vi "Three Button Dialog CORE.vi"(4 "Allow user to close window? (TRUE)":bool=TRUE caption="Darf Anwender das Fenster schließen? (WAHR)", 5 "Justify Message (Left)":enum16{"Left", "Center", "Right"}(ring) caption="Nachricht ausrichten (Links)", 6 "Keyboard Shortcuts (Left is <Enter>)":T1={"Left Button Key Shortcut"={"Control"=FALSE, "Shift"=FALSE, "Key"="<Enter>"}, "Center Button Key Shortcut"={"Control"=FALSE, "Shift"=FALSE, "Key"=""}, "Right Button Key Shortcut"={"Control"=FALSE, "Shift"=FALSE, "Key"=""}} caption="Tastenkombimationen (Links ist <Enter>)", 7 "Window Title (\"\")":string caption="Fenstertitel (\"\")", 8 "Right Button Text (\"Cancel\")":string="Abbrechen" caption="Text der rechten Schaltfläche (\"Abbrechen\")", 9 "Center Button Text (\"No\")":string="Nein" caption="Text für mittlere Maustaste (\"No\")", 10 "Left Button Text (\"Yes\")":string="Ja" caption="Text der linken Maustaste (\"Yes\")", 11 "message":string caption="Meldung") -> (3 "Which Button?":T2(ring)=enum."Center Button" caption="Welche Schaltfläche?")   [LabVIEW 2009]
doc: "Zeigt den Text in einem Dialog mit drei Schaltflächen an. Der Enum Ausgang gibt an welche der drei Schaltflächen ausgewählt wurde oder ob der Dialog ohne Auswahl abgebrochen wurde."
panel:
  in  "OK":string="OK"
  out "C-Message":string caption="C-Nachricht"
  in  "Right Button":bool caption="Rechte Schaltfläche"
  in  "Center Button":bool caption="Mittlere Schaltfläche"
  in  "Left Button":bool caption="Linke Schaltfläche"
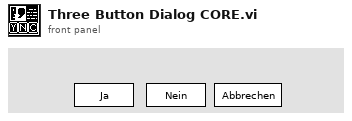
[diagram p1: front panel]
types:
  T1 = cluster{"Left Button Key Shortcut":cluster{"Control":bool, "Shift":bool, "Key":string}, "Center Button Key Shortcut":cluster{"Control":bool, "Shift":bool, "Key":string}, "Right Button Key Shortcut":cluster{"Control":bool, "Shift":bool, "Key":string}}
  T2 = enum16{"Left Button", "Center Button", "Right Button", "Window Close"}
  T3 = cluster{"left":i16, "top":i16, "right":i16, "bottom":i16}
  T4 = cluster{"Control":bool, "Shift":bool, "Key":string}
  T5 = typedef "LVRectTypeDef.ctl" = cluster{"left":i16, "top":i16, "right":i16, "bottom":i16}
  T6 = typedef "LVPointTypeDef.ctl" = cluster{"Horizontal":i16, "Vertical":i16}
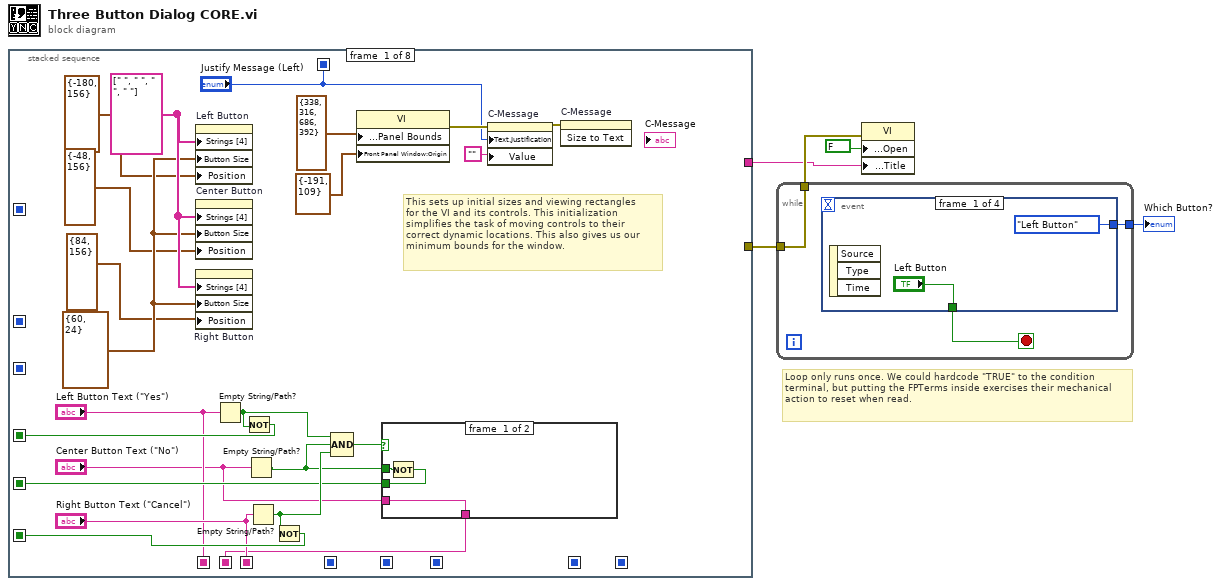
[diagram p0: block diagram]
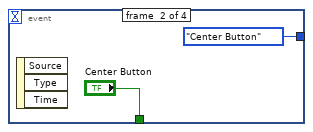
[diagram p2: hidden frame]
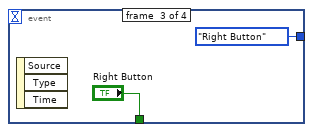
[diagram p3: hidden frame]
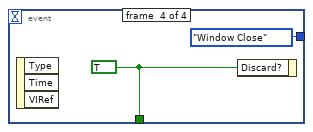
[diagram p4: hidden frame]
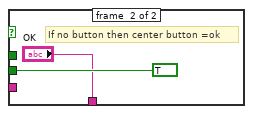
[diagram p5: hidden frame]
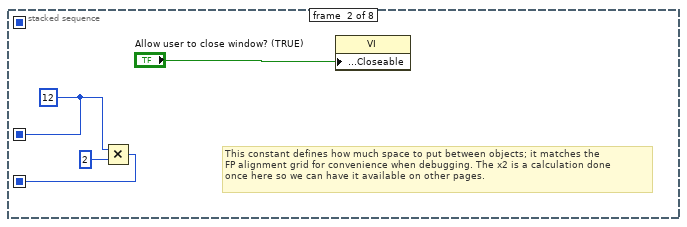
[diagram p6: hidden frame]
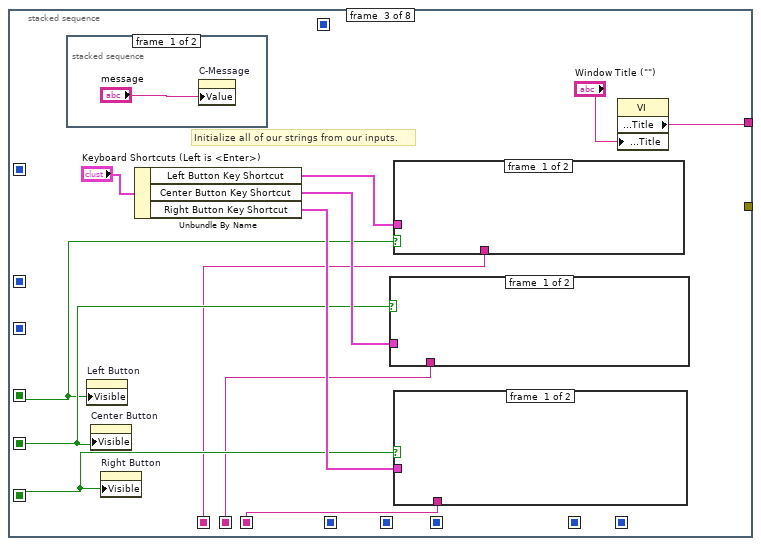
[diagram p7: hidden frame]
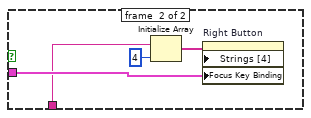
[diagram p8: hidden frame]
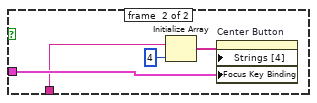
[diagram p9: hidden frame]
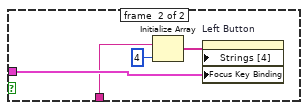
[diagram p10: hidden frame]
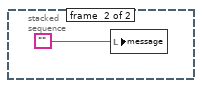
[diagram p11: hidden frame]
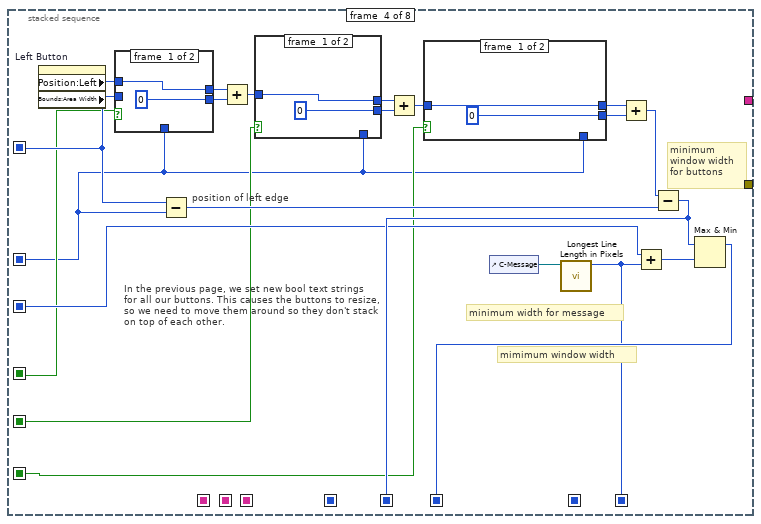
[diagram p12: hidden frame]
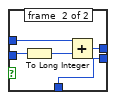
[diagram p13: hidden frame]
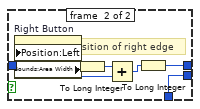
[diagram p14: hidden frame]
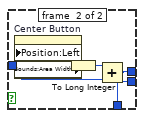
[diagram p15: hidden frame]
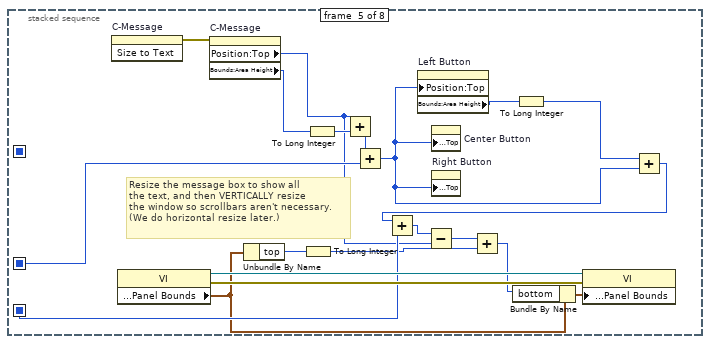
[diagram p16: hidden frame]
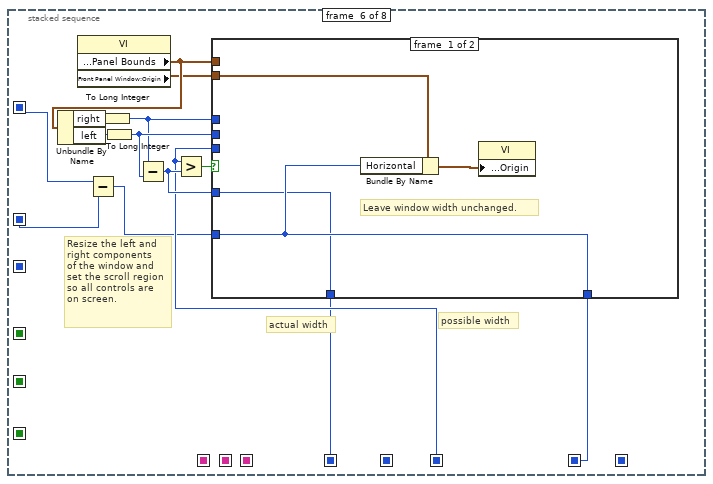
[diagram p17: hidden frame]
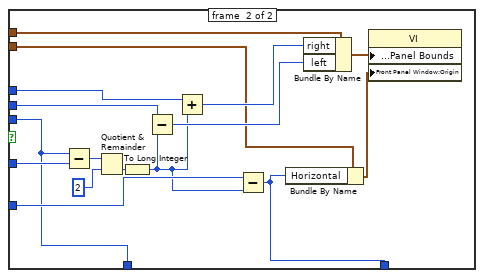
[diagram p18: hidden frame]
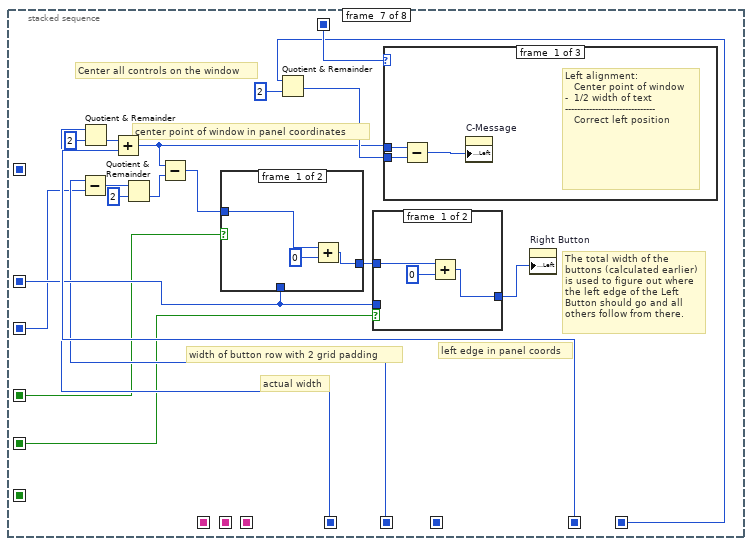
[diagram p19: hidden frame]
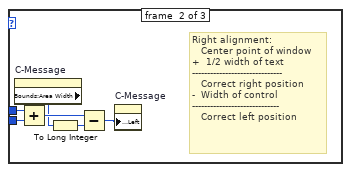
[diagram p20: hidden frame]
diagram:
  # "Loop only runs once. We could hardcode \"TRUE\" to the condition terminal, but putting the FPTerms inside exercises their mechanical action to reset when read."
  n1 = stacked-sequence {
    seq-local: [_ _ _ w83 _ _ _ _] -> [_ _ _ _ _ w139 _ _]
    seq-local: [_ _ _ _ _ w134 _ _] -> [_ _ _ _ _ _ w180 _]
    seq-local: [_ _ _ w80 _ _ _ _] -> [_ _ _ _ _ _ w173 _]
    seq-local: [_ _ _ w78 _ _ _ _] -> [_ _ _ _ _ w133 _ _]
    seq-local: [_ w36 _ _ _ _ _ _] -> [_ _ _ w65 w116 w132 w177 _]
    seq-local: [_ w34 _ _ _ _ _ _] -> [_ _ _ w79 w117 _ w172 _]
    seq-local: [_ _ _ _ _ w130 _ _] -> [_ _ _ _ _ _ w179 _]
    seq-local: [w13 _ _ _ _ _ _ _] -> [_ _ w42 w71 _ _ _ _]
    seq-local: [w16 _ _ _ _ _ _ _] -> [_ _ w41 w73 _ _ w166 _]
    seq-local: [w14 _ _ _ _ _ _ _] -> [_ _ w40 w69 _ _ w167 _]
    seq-local: ["Left Button Text (\"Yes\")" _ _ _ _ _ _ _] -> [_ _ w39 _ _ _ _ _]
    seq-local: [w7 _ _ _ _ _ _ _] -> [_ _ w38 _ _ _ _ _]
    seq-local: ["Right Button Text (\"Cancel\")" _ _ _ _ _ _ _] -> [_ _ w37 _ _ _ _ _]
    seq-local: [_ _ _ w63 _ _ _ _] -> [_ _ _ _ _ _ w163 _]
    seq-local: ["Justify Message (Left)" _ _ _ _ _ _ _] -> [_ _ _ _ _ _ w164 _]
    tunnel: [_ _ _ _ _ _ _ w214] -> w3
    tunnel: [_ _ w46 _ _ _ _ _] -> w1
    frame #0 {
      w27 = string[] [" ", " ", " ", " "] ("Strings [4]")
      w26 = cluster{"Width":u32, "Height":u32} {"Width"=60, "Height"=24} ("Button Size")
      # "This sets up initial sizes and viewing rectangles\nfor the VI and its controls. This initialization\nsimplifies the task of moving controls to their\ncorrect dynamic locations. This also gives us our\nminimum bounds for the window."
      n2 = property on="Left Button" class="Boolean"("Strings [4]"=w27, "Button Size"=w26, "Position"=cluster{"Left":i32, "Top":i32} {"Left"=-180, "Top"=156}) -> ()  [unwired: 2 in, 2 out]
      n3 = property on="Center Button" class="Bool"("Strings [4]"=w27, "Button Size"=w26, "Position"=cluster{"Left":i32, "Top":i32} {"Left"=-48, "Top"=156}) -> ()  [unwired: 2 in, 2 out]
      n4 = property on="Right Button" class="Bool"("Strings [4]"=w27, "Button Size"=w26, "Position"=cluster{"Left":i32, "Top":i32} {"Left"=84, "Top"=156}) -> ()  [unwired: 2 in, 2 out]
      n5 = Empty String/Path?(string/path="Left Button Text (\"Yes\")") -> (empty?=w19:bool)
      n6 = Not(x=w19) -> (.not. x?=w14:bool)
      n7 = Empty String/Path?(string/path="Center Button Text (\"No\")") -> (empty?=w15:bool)
      n8 = Empty String/Path?(string/path="Right Button Text (\"Cancel\")") -> (empty?=w18:bool)
      n9 = Not(x=w18) -> (.not. x?=w13:bool)
      n10 = Compound Arithmetic op=AND(w19, w15, w18) -> (w17:bool)
      n11 = property class="VI"("Front Panel Window:Panel Bounds"=T3 {"left"=338, "top"=316, "right"=686, "bottom"=392} ("Front Panel.PanelBounds"), "Front Panel Window:Origin"=cluster{"Horizontal":i16, "Vertical":i16} {"Horizontal"=-191, "Vertical"=109} ("Front Panel.Origin")) -> (error out=w21:errorcluster)  [unwired: 2 in, 1 out]
      n12 = case shown="True" w17 {
        tunnel: w15 -> [w30 _]
        tunnel: [w29 TRUE] -> w16
        tunnel: "Center Button Text (\"No\")" -> [w28 _]
        tunnel: [w28 "OK"] -> w7
        frame #0 {
          n13 = Not(x=w30) -> (.not. x?=w29:bool)
        }
        frame #1 {
          # "If no button then center button =ok"
        }
      }
      n14 = property on="C-Message" class="Str"(error in=w21, "Text.Justification"="Justify Message (Left)", "Value"="") -> (error out=w20:errorcluster)  [unwired: 1 in, 1 out]
      n15 = invoke on="C-Message" class="Str" method="Size to Text"(error in=w20) -> ()  [unwired: 2 in, 3 out]
    }
    frame #1 {
      w36 = 12 ("grid spacing")
      # "This constant defines how much space to put between objects; it matches the \nFP alignment grid for convenience when debugging. The x2 is a calculation done\nonce here so we can have it available on other pages."
      n16 = Multiply(x=w36, y=2) -> (x*y=w34:i32)
      n17 = property class="VI"("Front Panel Window:Closeable"="Allow user to close window? (TRUE)") -> ()  [unwired: 2 in, 2 out]
    }
    frame #2 {
      # "Initialize all of our strings from our inputs."
      n18 = stacked-sequence {
        frame #0 {
          n19 = property on="C-Message" class="Str"("Value"="message") -> ()  [unwired: 2 in, 2 out]
        }
        frame #1 {
          n20 = local write "message"("") -> ()
        }
      }
      n21 = property on="Left Button" class="Boolean"("Visible"=w40) -> ()  [unwired: 2 in, 2 out]
      n22 = property on="Center Button" class="Bool"("Visible"=w41) -> ()  [unwired: 2 in, 2 out]
      n23 = property on="Right Button" class="Bool"("Visible"=w42) -> ()  [unwired: 2 in, 2 out]
      n24 = Unbundle By Name("Keyboard Shortcuts (Left is <Enter>)") -> ("Left Button Key Shortcut"=w43:T4, "Center Button Key Shortcut"=w44:T4, "Right Button Key Shortcut"=w45:T4)
      n25 = case shown="True" w41 {
        tunnel: w44 -> [_ w54]
        tunnel: w38 -> [_ w53]
        frame #0 {
        }
        frame #1 {
          n26 = Initialize Array(w53, 4 ("dimension size")) -> (w56:string[])
          n27 = property on="Center Button" class="Bool"("Strings [4]"=w56, "Focus Key Binding"=w54) -> ()  [unwired: 2 in, 2 out]
        }
      }
      n28 = case shown="True" w40 {
        tunnel: w43 -> [_ w58]
        tunnel: w39 -> [_ w57]
        frame #0 {
        }
        frame #1 {
          n29 = Initialize Array(w57, 4 ("dimension size")) -> (w60:string[])
          n30 = property on="Left Button" class="Boolean"("Strings [4]"=w60, "Focus Key Binding"=w58) -> ()  [unwired: 2 in, 2 out]
        }
      }
      n31 = case shown="True" w42 {
        tunnel: w45 -> [_ w50]
        tunnel: w37 -> [_ w49]
        frame #0 {
        }
        frame #1 {
          n32 = Initialize Array(w49, 4 ("dimension size")) -> (w52:string[])
          n33 = property on="Right Button" class="Bool"("Strings [4]"=w52, "Focus Key Binding"=w50) -> ()  [unwired: 2 in, 2 out]
        }
      }
      n34 = property class="VI"("Front Panel Window:Title"="Window Title (\"\")") -> ("Front Panel Window:Title"=w46:string)  [unwired: 2 in, 2 out]
    }
    frame #3 {
      # "In the previous page, we set new bool text strings\nfor all our buttons. This causes the buttons to resize,\nso we need to move them around so they don't stack\non top of each other."
      # "mimimum window width"
      # "minimum width for message"
      # "minimum\nwindow width\nfor buttons"
      # "position of left edge"
      n35 = property on="Left Button" class="Boolean"() -> ("Position:Left"=w78:i32, "Bounds:Area Width"=w75:u32)  [unwired: 2 in, 2 out]
      n36 = case shown="True" w69 {
        tunnel: w78 -> [w86 w91]
        tunnel: w75 -> [_ w90]
        tunnel: [w86 w89] -> w70
        tunnel: w65 -> [_ w87]
        tunnel: [0 w87] -> w68
        frame #0 {
        }
        frame #1 {
          n37 = To Long Integer(number=w90) -> (32bit integer=w88:i32)
          n38 = Add(x=w91, y=w88) -> (x+y=w89:i32)
        }
      }
      n39 = Subtract(x=w78, y=w65) -> (x-y=w81:i32)
      n40 = Add(x=w70, y=w68) -> (x+y=w76:i32)
      n41 = case shown="True" w73 {
        tunnel: w76 -> [w101 w106]
        tunnel: [w101 w105] -> w74
        tunnel: [0 w102] -> w67
        tunnel: w65 -> [_ w102]
        frame #0 {
        }
        frame #1 {
          n42 = property on="Center Button" class="Bool"("Position:Left"=w106) -> ("Bounds:Area Width"=w104:u32)  [unwired: 2 in, 2 out]
          n43 = To Long Integer(number=w104) -> (32bit integer=w103:i32)
          n44 = Add(x=w103, y=w106) -> (x+y=w105:i32)
        }
      }
      n45 = Add(x=w74, y=w67) -> (x+y=w77:i32)
      n46 = case shown="True" w71 {
        tunnel: w77 -> [w93 w99]
        tunnel: [w93 w97] -> w72
        tunnel: [0 w94] -> w66
        tunnel: w65 -> [_ w94]
        frame #0 {
        }
        frame #1 {
          # "position of right edge"
          n47 = property on="Right Button" class="Bool"("Position:Left"=w99) -> ("Bounds:Area Width"=w96:u32)  [unwired: 2 in, 2 out]
          n48 = To Long Integer(number=w96) -> (32bit integer=w95:i32)
          n49 = Add(x=w95, y=w99) -> (x+y=w98:i32)
          n50 = To Long Integer(number=w98) -> (32bit integer=w97:i32)
        }
      }
      n51 = control-ref of="C-Message"() -> (w64:refnum<vi>)
      n52 = call "Longest Line Length in Pixels.vi"("String"=w64) -> ("longest line length"=w63:i32)  [unwired: 9 in]
      n53 = Add(x=w72, y=w66) -> (x+y=w82:i32)
      n54 = Add(x=w79, y=w63) -> (x+y=w84:i32)
      n55 = Subtract(x=w82, y=w81) -> (x-y=w80:i32)
      n56 = Max & Min(x=w80, y=w84) -> (max(x,y)=w83:i32)  [unwired: 1 out]
    }
    frame #4 {
      # "Resize the message box to show all\nthe text, and then VERTICALLY resize\nthe window so scrollbars aren't necessary.\n(We do horizontal resize later.)"
      n57 = invoke on="C-Message" class="Str" method="Size to Text"() -> (error out=w109:errorcluster)  [unwired: 3 in, 2 out]
      n58 = property class="VI"() -> (reference out=w124:refnum<vi>, error out=w125:errorcluster, "Front Panel Window:Panel Bounds"=w113:T5)  [unwired: 2 in]
      n59 = property on="C-Message" class="Str"(error in=w109) -> ("Position:Top"=w108:i32, "Bounds:Area Height"=w107:u32)  [unwired: 1 in, 2 out]
      n60 = Unbundle By Name(w113) -> ("top"=w122:i16)
      n61 = To Long Integer(number=w122) -> (32bit integer=w114:i32)
      n62 = To Long Integer(number=w107) -> (32bit integer=w115:i32)
      n63 = Add(x=w108, y=w115) -> (x+y=w118:i32)
      n64 = Add(x=w118, y=w116) -> (x+y=w111:i32)
      n65 = property on="Left Button" class="Boolean"("Position:Top"=w111) -> ("Bounds:Area Height"=w112:u32)  [unwired: 2 in, 2 out]
      n66 = property on="Center Button" class="Bool"("Position:Top"=w111) -> ()  [unwired: 2 in, 2 out]
      n67 = property on="Right Button" class="Bool"("Position:Top"=w111) -> ()  [unwired: 2 in, 2 out]
      n68 = To Long Integer(number=w112) -> (32bit integer=w110:i32)
      n69 = Add(x=w110, y=w111) -> (x+y=w119:i32)
      n70 = Add(x=w119, y=w117) -> (x+y=w120:i32)
      n71 = Subtract(x=w120, y=w108) -> (x-y=w123:i32)
      n72 = Add(x=w123, y=w114) -> (x+y=w121:i32)
      n73 = Bundle By Name(cluster=w113, "bottom"=w121) -> (w126:T5)
      n74 = property class="VI"(reference=w124, error in=w125, "Front Panel Window:Panel Bounds"=w126) -> ()  [unwired: 2 out]
    }
    frame #5 {
      # "Resize the left and\nright components\nof the window and\nset the scroll region\nso all controls are \non screen."
      # "actual width"
      # "possible width"
      n75 = property class="VI"() -> ("Front Panel Window:Panel Bounds"=w136:T5, "Front Panel Window:Origin"=w129:T6)  [unwired: 2 in, 2 out]
      n76 = Unbundle By Name(w136) -> ("right"=w138:i16, "left"=w137:i16)
      n77 = Subtract(x=w133, y=w132) -> (x-y=w131:i32)
      n78 = To Long Integer(number=w138) -> (32bit integer=w127:i32)
      n79 = To Long Integer(number=w137) -> (32bit integer=w128:i32)
      n80 = Subtract(x=w127, y=w128) -> (x-y=w140:i32)
      n81 = Greater?(x=w139, y=w140) -> (0:w135:bool)
      n82 = case shown="True" w135 {
        tunnel: w140 -> [w141 w160]
        tunnel: w139 -> [_ w146]
        tunnel: w127 -> [_ w155]
        tunnel: w128 -> [_ w156]
        tunnel: w136 -> [_ w157]
        tunnel: [w144 w148] -> w134
        tunnel: w129 -> [w142 w150]
        tunnel: w131 -> [w144 w147]
        tunnel: [w141 w146] -> w130
        frame #0 {
          # "Leave window width unchanged."
          n83 = Bundle By Name(cluster=w142, "Horizontal"=w144) -> (w143:T6)
          n84 = property class="VI"("Front Panel Window:Origin"=w143) -> ()  [unwired: 2 in, 2 out]
        }
        frame #1 {
          n85 = Subtract(x=w146, y=w160) -> (x-y=w159:i32)
          n86 = Quotient & Remainder(x=w159, y=2) -> (floor(x/y)=w152:i32)  [unwired: 1 out]
          n87 = To Long Integer(number=w152) -> (32bit integer=w145:i32)
          n88 = Subtract(x=w156, y=w145) -> (x-y=w153:i32)
          n89 = Add(x=w155, y=w145) -> (x+y=w154:i32)
          n90 = Subtract(x=w147, y=w145) -> (x-y=w148:i32)
          n91 = Bundle By Name(cluster=w150, "Horizontal"=w148) -> (w149:T6)
          n92 = Bundle By Name(cluster=w157, "right"=w154, "left"=w153) -> (w151:T5)
          n93 = property class="VI"("Front Panel Window:Panel Bounds"=w151, "Front Panel Window:Origin"=w149) -> ()  [unwired: 2 in, 2 out]
        }
      }
    }
    frame #6 {
      # "The total width of the buttons (calculated earlier) is used to figure out where the left edge of the Left Button should go and all others follow from there."
      # "left edge in panel coords"
      # "actual width"
      # "width of button row with 2 grid padding"
      # "center point of window in panel coordinates"
      # "Center all controls on the window"
      n94 = Subtract(x=w173, y=w172) -> (x-y=w174:i32)
      n95 = Quotient & Remainder(x=w179, y=2) -> (floor(x/y)=w176:i32)  [unwired: 1 out]
      n96 = Add(x=w176, y=w180) -> (x+y=w161:i32)
      n97 = Quotient & Remainder(x=w174, y=2) -> (floor(x/y)=w171:i32)  [unwired: 1 out]
      n98 = Subtract(x=w161, y=w171) -> (x-y=w170:i32)
      n99 = case shown="True" w167 {
        tunnel: w177 -> [_ w211]
        tunnel: w170 -> [w206 w210]
        tunnel: [w205 w208] -> w169
        frame #0 {
          n100 = Add(x=w206, y=0) -> (x+y=w205:i32)
        }
        frame #1 {
          n101 = property on="Left Button" class="Bool"("Position:Left"=w210) -> ("Bounds:Area Width"=w209:u32)  [unwired: 2 in, 2 out]
          n102 = To Long Integer(number=w209) -> (32bit integer=w207:i32)
          n103 = Compound Arithmetic op=ADD(w207, w210, w211) -> (w208:i32)
        }
      }
      n104 = Quotient & Remainder(x=w163, y=2) -> (floor(x/y)=w162:i32)  [unwired: 1 out]
      n105 = case shown="True" w166 {
        tunnel: w177 -> [_ w203]
        tunnel: w169 -> [w198 w201]
        tunnel: [w197 w200] -> w168
        frame #0 {
          n106 = Add(x=w198, y=0) -> (x+y=w197:i32)
        }
        frame #1 {
          n107 = property on="Center Button" class="Bool"("Position:Left"=w201) -> ("Bounds:Area Width"=w202:u32)  [unwired: 2 in, 2 out]
          n108 = To Long Integer(number=w202) -> (32bit integer=w199:i32)
          n109 = Compound Arithmetic op=ADD(w199, w201, w203) -> (w200:i32)
        }
      }
      n110 = case shown="\"Right\"" w164 {
        tunnel: w161 -> [w183 w189 w191]
        tunnel: w162 -> [w181 w188 _]
        frame #0 {
          # "Left alignment:\n   Center point of window\n-  1/2 width of text\n------------------------------\n   Correct left position"
          n111 = Subtract(x=w183, y=w181) -> (x-y=w182:i32)
          n112 = property on="C-Message" class="Str"("Position:Left"=w182) -> ()  [unwired: 2 in, 2 out]
        }
        frame #1 {
          # "Right alignment:\n   Center point of window\n+  1/2 width of text\n------------------------------\n   Correct right position\n-  Width of control\n-----------------------------\n   Correct left position"
          n113 = property on="C-Message" class="Str"() -> ("Bounds:Area Width"=w185:u32)  [unwired: 2 in, 2 out]
          n114 = Add(x=w189, y=w188) -> (x+y=w187:i32)
          n115 = To Long Integer(number=w185) -> (32bit integer=w184:i32)
          n116 = Subtract(x=w187, y=w184) -> (x-y=w186:i32)
          n117 = property on="C-Message" class="Str"("Position:Left"=w186) -> ()  [unwired: 2 in, 2 out]
        }
        frame #2 {
          # "Center alignment:\n   Center point of window\n-  1/2 width of control\n------------------------------\n   Correct left position\n\n(the text is itself centered in the control, so centering control centers text)"
          n118 = property on="C-Message" class="Str"() -> ("Bounds:Area Width"=w194:u32)  [unwired: 2 in, 2 out]
          n119 = To Long Integer(number=w194) -> (32bit integer=w192:i32)
          n120 = Quotient & Remainder(x=w192, y=2) -> (floor(x/y)=w190:i32)  [unwired: 1 out]
          n121 = Subtract(x=w191, y=w190) -> (x-y=w193:i32)
          n122 = property on="C-Message" class="Str"("Position:Left"=w193) -> ()  [unwired: 2 in, 2 out]
        }
      }
      n123 = property on="Right Button" class="Bool"("Position:Left"=w168) -> ()  [unwired: 2 in, 2 out]
    }
    frame #7 {
      w212 = TRUE ("Front Panel Window:Open")
      # "Center the window itself and put it on screen."
      n124 = property class="VI"("Front Panel Window:Auto Center (Deprecated)"=FALSE ("Front Panel Window:Auto Center"), "Front Panel Window:Auto Center (Deprecated)"=w212, "Front Panel Window:Open"=w212) -> (error out=w214:errorcluster)  [unwired: 2 in, 1 out]
    }
  }
  n125 = while {
    tunnel: [w217] -> w4
    tunnel: [w216] -> w2
    tunnel: w3 -> [w216]
    stop <- w215 stop-if-true
    n126 = event shown="[3] Panel Close?" {
      selector: _ -> [_ _ _ _]
      dyn-events: _ -> [_ _ _ _]
      timeout: _ -> [_ _ _ _]
      tunnel: ["Left Button" "Center Button" "Right Button" w224] -> w215
      tunnel: [T2."Left Button" ("Which Button?") T2."Center Button" ("Which Button?") T2."Right Button" ("Which Button?") T2."Window Close" ("Which Button?")] -> w217
      event #0 {
        n127 = event-data() -> ()  [unwired: 1 in, 3 out]
      }
      event #1 {
        n128 = event-data() -> ()  [unwired: 1 in, 3 out]
      }
      event #2 {
        n129 = event-data() -> ()  [unwired: 1 in, 3 out]
      }
      event #3 {
        w224 = TRUE ("Discard?")
        n130 = event-data() -> ()  [unwired: 1 in, 3 out]
        n131 = event-data("Discard?"=w224) -> ()  [unwired: 1 in, 1 out]
      }
    }
  }
  "Which Button?" <- w4
  n132 = property class="VI"(error in=w2, "Front Panel Window:Open"=FALSE, "Front Panel Window:Title"=w1) -> ()  [unwired: 1 in, 2 out]
